vi "AlliGator Load IRFs & Fit Data (Map) HDF5 File v0.3.vi"(8 "Error In":errorcluster, 9 "File Type & Version only":bool, 11 "File Path":path) -> (0 "error out":errorcluster, 1 "Data Description":string, 2 "Decay Fit Options & Parameters":T1 {"Fit Options"."Offset Resolution" min=0.0; "Fit Options"."Period" min=0.0; "Fit Options"."Min Decay Percentile" min=0.0 max=1.0; "Fit Options"."Max Decay Percentile" min=0.0 max=100.0; "Fit Parameter Constraints"."Max Value" format="%#.3g"; "Fit Parameter Constraints"."Min Value" format="%#.3g"}, 3 "IRFs & Fit Data Map":T13 {"Fit Options: Decay Preprocessing Parameters"."# Folds" min=1}, 4 "[Multiple Decays Fit Parameters SDV]":dbl[][](array[numeric]), 5 "File Version":string, 7 "File Type":string)   [LabVIEW 2021, in "AlliGator Decay Fit Parameter Map.lvlib"]
doc: "Loads Decay Fit Parameter Map and associated metadata."
uses:
  AlliGator Decay Fit Parameter Map.lvlib
  AlliGator IRFs & Fit Data v2.ctl
  Fits/IRF(X)PSED/Decay Fit Parameters & Derived Quantities List.ctl
  AlliGator Decay Preprocessing Parameters.ctl
  Graphs/XY Graph/XY Graph Plot Shift Parameters.ctl
  Graphs/XY Graph/XY Graph Plot Shift Method.ctl
  AlliGator Decay Fit Options & Parameters v2.ctl
  Fits/IRF(X)PSED/Decay Fit Options v2.ctl
  Fits/Decay Convolution/Decay Model.ctl
  Fits/Residual Type.ctl
  Fits/IRF(X)PSED/Fit Weights Type.ctl
  Fits/Non-linear Fitting Method v2.ctl
  Fits/Fit Calculation Method.ctl
  Fits/Non-linear Fitting Algorithm.ctl
  AlliGator Decay Fit Parameter Constraints 2.ctl
  Fits/IRF(X)PSED/Decay Fit Parameters In List.ctl
  Fits/IRF(X)PSED/MLE Baseline Offset Type.ctl
  Fits/IRF(X)PSED/Decay Fit Options v1.ctl
  Fits/Non-linear Fitting Method v1.ctl
  AlliGator IRFs & Fit Data v1.ctl
  AlliGator Decay Fit Options & Parameters v1.ctl
  <vilib>/addons/h5labview2/base/lib_path.vi
  <vilib>/addons/h5labview2/base/H5Equery.vi
  <vilib>/addons/h5labview2/base/hid_t.ctl
  <vilib>/addons/h5labview2/dataset/H5Dread.llb/H5Dread.xnode
  <vilib>/addons/h5labview2/file/H5F.lvlib
  <vilib>/addons/h5labview2/group/H5G.lvlib
  Time/Time.lvlib
  Fits/Fits.lvlib
  Strings/Strings.lvlib
  AlliGator Decay Fit.lvlib
  Graphs/XY Graph/XY Graph Add-Ons.lvlib
  AlliGator Decay Preprocessing.lvlib
panel:
  in  "Fit Parameter":T12(ring)
  out "elapsed (relative) seconds":dbl
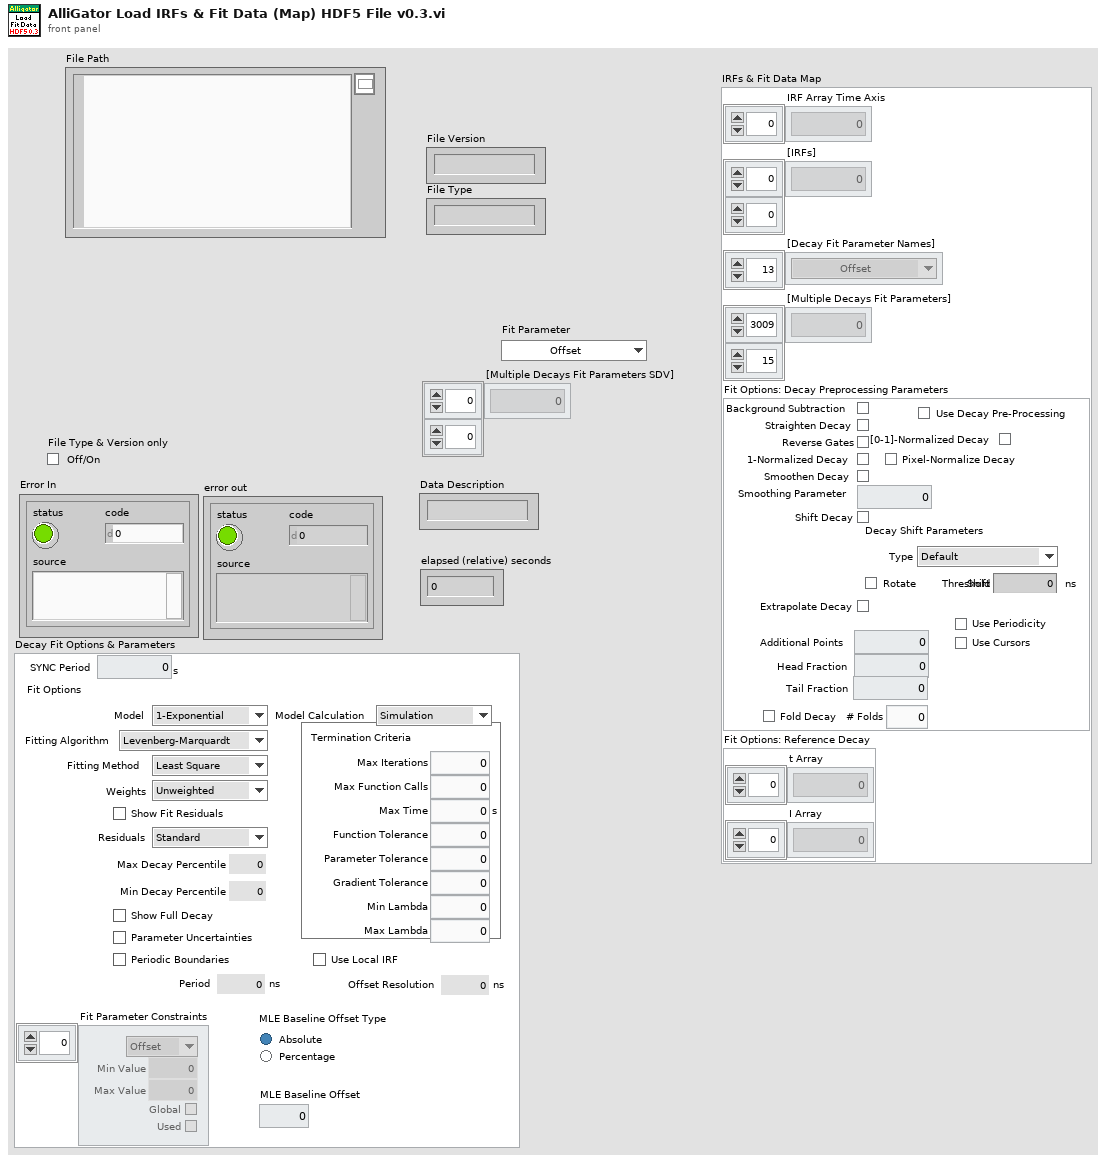
[diagram p1: front panel]
types:
  T1 = typedef "AlliGator Decay Fit Parameter Map.lvlib/AlliGator Decay Fit Options & Parameters v2.ctl" = cluster{"SYNC Period":dbl[unit], "Fit Options":T2, "Fit Parameter Constraints":T9[], "MLE Baseline Offset":dbl, "MLE Baseline Offset Type":T11}
  T2 = typedef "Fits.lvlib/Decay Fit Options v2.ctl" = cluster{"Show Fit Residuals":bool, "Fit Model":T3, "Residual Type":T4, "Max Decay Percentile":dbl, "Min Decay Percentile":dbl, "Show Full Decay":bool, "Weights":T5, "Fitting Method":T6, "Compute Parameter Uncertainties":bool, "Periodic Boundaries":bool, "Model Calculation":T7, "Period":dbl[unit], "Termination Criteria":cluster{"Max Iterations":i32, "Max Function Calls":i32, "Max Time":dbl[unit], "Function Tolerance":dbl, "Parameter Tolerance":dbl, "Gradient Tolerance":dbl, "Min Lambda":dbl, "Max Lambda":dbl, "Initial Tick Count":u32}, "Offset Resolution":dbl[unit], "Use Local IRF":bool, "Fitting Algorithm":T8}
  T3 = typedef "Fits.lvlib/Decay Model.ctl" = enum16{"1-Exponential", "2-Exponentials"}
  T4 = typedef "Fits.lvlib/Residual Type.ctl" = enum16{"Standard", "Normalized", "Reduced"}
  T5 = typedef "Fits.lvlib/Fit Weights Type.ctl" = enum16{"Unweighted", "1/Variance", "Best of All"}
  T6 = typedef "Fits.lvlib/Non-linear Fitting Method v2.ctl" = enum16{"Least Square", "Least Absolute Residual", "Bisquare", "MLE", "-", "Best of All"}
  T7 = typedef "Fits.lvlib/Fit Calculation Method.ctl" = enum16{"Simulation", "Convolution", "Integration"}
  T8 = typedef "Fits.lvlib/Non-linear Fitting Algorithm.ctl" = enum16{"Levenberg-Marquardt", "Trust-Region Dogleg"}
  T9 = typedef "AlliGator Decay Analysis.lvlib/AlliGator Decay Fit.lvlib/AlliGator Decay Fit Parameter Constraints 2.ctl" = cluster{"Fit Parameter":T10, "Min Value":dbl, "Max Value":dbl, "Global":bool, "Used":bool}
  T10 = typedef "Fits.lvlib/Decay Fit Parameters In List.ctl" = enum16{"Offset", "Baseline", "A_1", "tau_1", "A_2", "tau_2"}
  T11 = typedef "Fits.lvlib/MLE Baseline Offset Type.ctl" = enum32{"Absolute", "Percentage"}
  T12 = enum16{"Offset", "Baseline", "A_1", "tau_1", "A_2", "tau_2", "<tau>_1", "f1_1", "f2_1", "<tau>_2", "f1_2", "f2_2", "-", "R^2", "Chi^2"}
  T13 = typedef "AlliGator Decay Fit Parameter Map.lvlib/AlliGator IRFs & Fit Data v2.ctl" = cluster{"IRF Array Time Axis":dbl[], "[IRFs]":dbl[][], "[Decay Fit Parameter Names]":T14[], "[Multiple Decays Fit Parameters]":dbl[][], "Fit Options: Decay Preprocessing Parameters":T15, "Fit Options: Reference Decay":cluster{"t Array":dbl[], "I Array":dbl[]}}
  T14 = typedef "Fits.lvlib/Decay Fit Parameters & Derived Quantities List.ctl" = enum16{"Offset", "Baseline", "A_1", "tau_1", "A_2", "tau_2", "<tau>_a", "f1_a", "f2_a", "<tau>_i", "f1_i", "f2_i", "-", "R^2", "Chi^2"}
  T15 = typedef "AlliGator Decay Analysis.lvlib/AlliGator Decay Preprocessing.lvlib/AlliGator Decay Preprocessing Parameters.ctl" = cluster{"Background Subtraction":bool, "Straighten Decay":bool, "Reverse Gates":bool, "1-Normalized Decay":bool, "Smoothen Decay":bool, "Smoothing Parameter":dbl, "Shift Decay":bool, "Decay Shift Parameters":T16, "Extrapolate Decay":bool, "Additional Points":u32, "Head Fraction":dbl, "Pixel-Normalize Decay":bool, "Use Periodicity":bool, "Use Cursors":bool, "Tail Fraction":dbl, "Use Decay Pre-Processing":bool, "Fold Decay":bool, "# Folds":u32, "[0-1]-Normalized Decay":bool}
  T16 = typedef "XY Graph Add-Ons.lvlib/XY Graph Plot Shift Parameters.ctl" = cluster{"Type":T17, "Shift":dbl[unit], "Threshold":dbl, "Rotate":bool}
  T17 = typedef "XY Graph Add-Ons.lvlib/XY Graph Plot Shift Method.ctl" = enum16{"Default", "CFD", "Threshold", "Cross-Correlation"}
  T18 = typedef "AlliGator Decay Analysis.lvlib/AlliGator Decay Fit.lvlib/AlliGator Decay Fit Options & Parameters v1.ctl" = cluster{"SYNC Period":dbl[unit], "Fit Options":T19, "Fit Parameter Constraints":T9[]}
  T19 = typedef "Fits.lvlib/Decay Fit Options v1.ctl" = cluster{"Show Fit Residuals":bool, "Fit Model":T3, "Residual Type":T4, "Max Decay Percentile":dbl, "Min Decay Percentile":dbl, "Show Full Decay":bool, "Weights":T5, "Fitting Method":T20, "Compute Parameter Uncertainties":bool, "Periodic Boundaries":bool, "Model Calculation":T7, "Period":dbl[unit], "Termination Criteria":cluster{"Max Iterations":i32, "Max Function Calls":i32, "Max Time":dbl[unit], "Function Tolerance":dbl, "Parameter Tolerance":dbl, "Gradient Tolerance":dbl, "Min Lambda":dbl, "Max Lambda":dbl, "Initial Tick Count":u32}, "Offset Resolution":dbl[unit], "Use Local IRF":bool, "Fitting Algorithm":T8}
  T20 = typedef "Fits.lvlib/Non-linear Fitting Method v1.ctl" = enum16{"Least Square", "Least Absolute Residual", "Bisquare", "-", "Best of All"}
  T21 = typedef "AlliGator Decay Fit Parameter Map.lvlib/AlliGator IRFs & Fit Data v1.ctl" = cluster{"IRF Array Time Axis":dbl[], "[IRF]":dbl[][], "[Decay Fit Parameter Name]":T14[], "[Multiple Decays Fit Parameters]":dbl[][]}
  T22 = typedef "hid_t.ctl" = i64
  T23 = cluster{"Laser Period":dbl[unit], "Fit Options":T19, "Fit Parameter Constraints":T9[]}
  T24 = cluster{"IRF Array Time Axis":dbl[], "[IRF]":dbl[][], "[Decay Fit Parameter Name]":T14[], "[Multiple Decays Fit Parameters]":dbl[][]}
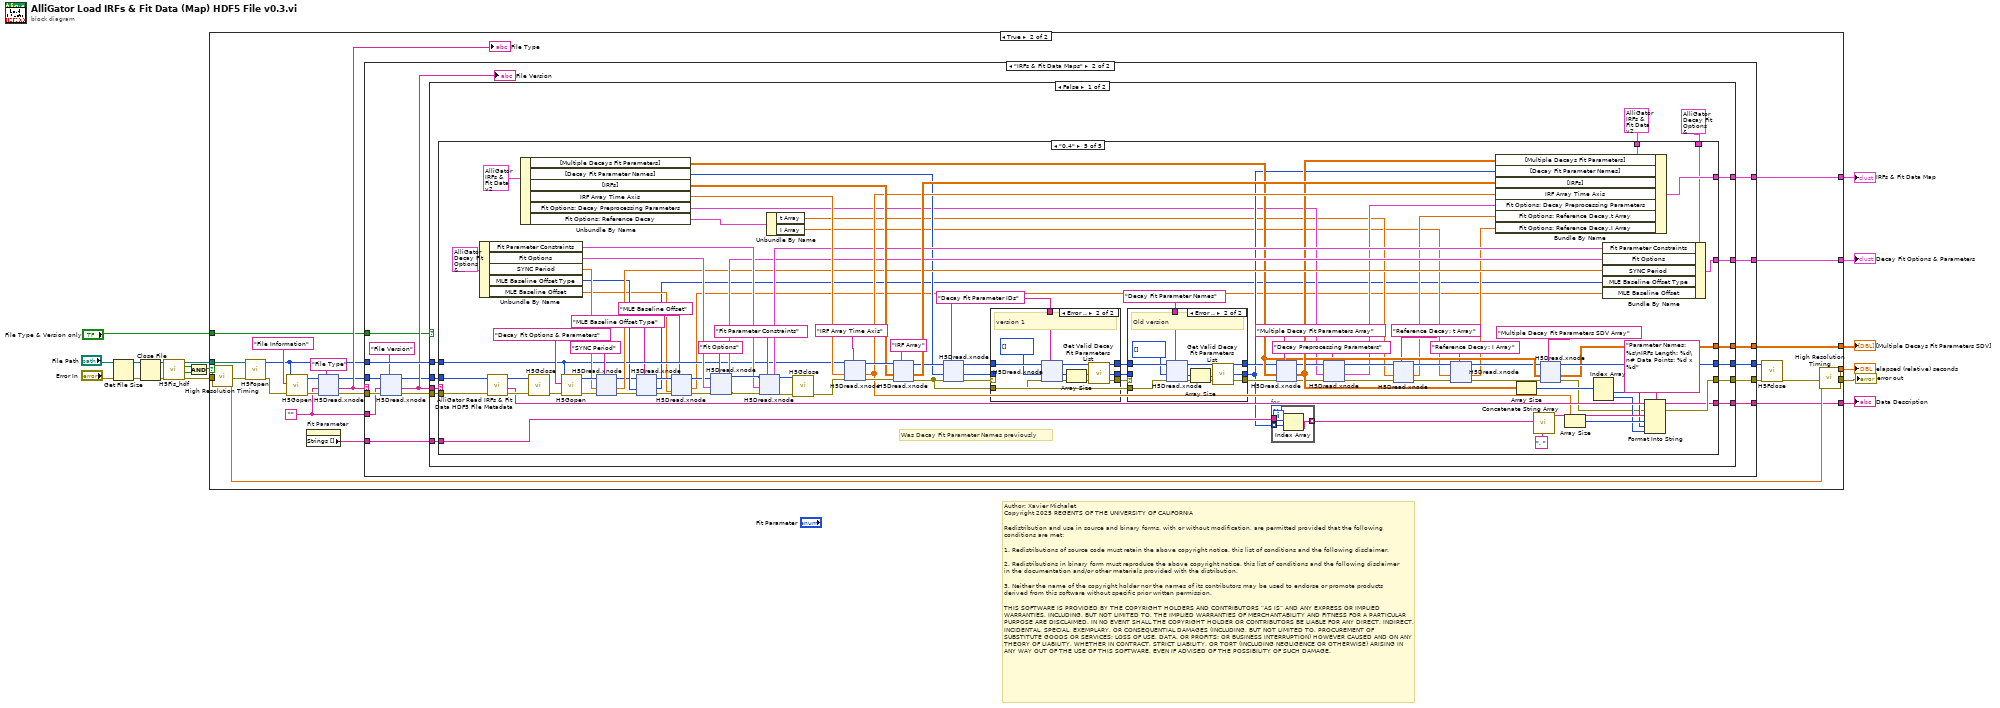
[diagram p0: block diagram]
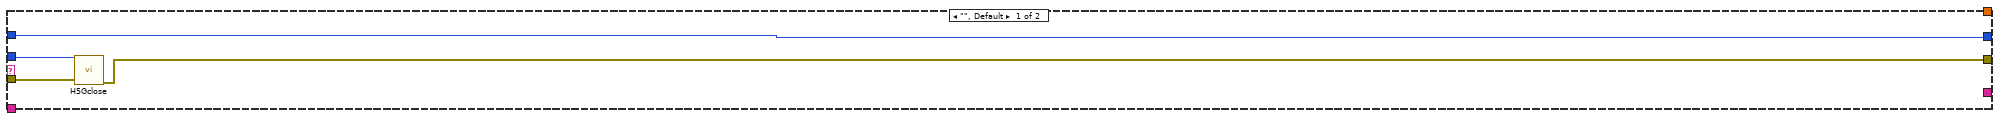
[diagram p3: hidden frame]
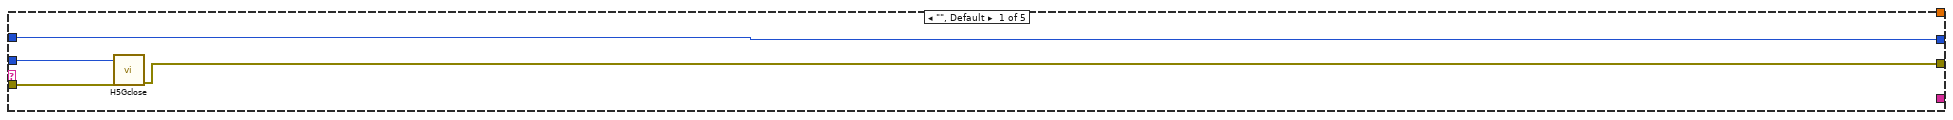
[diagram p4: hidden frame]
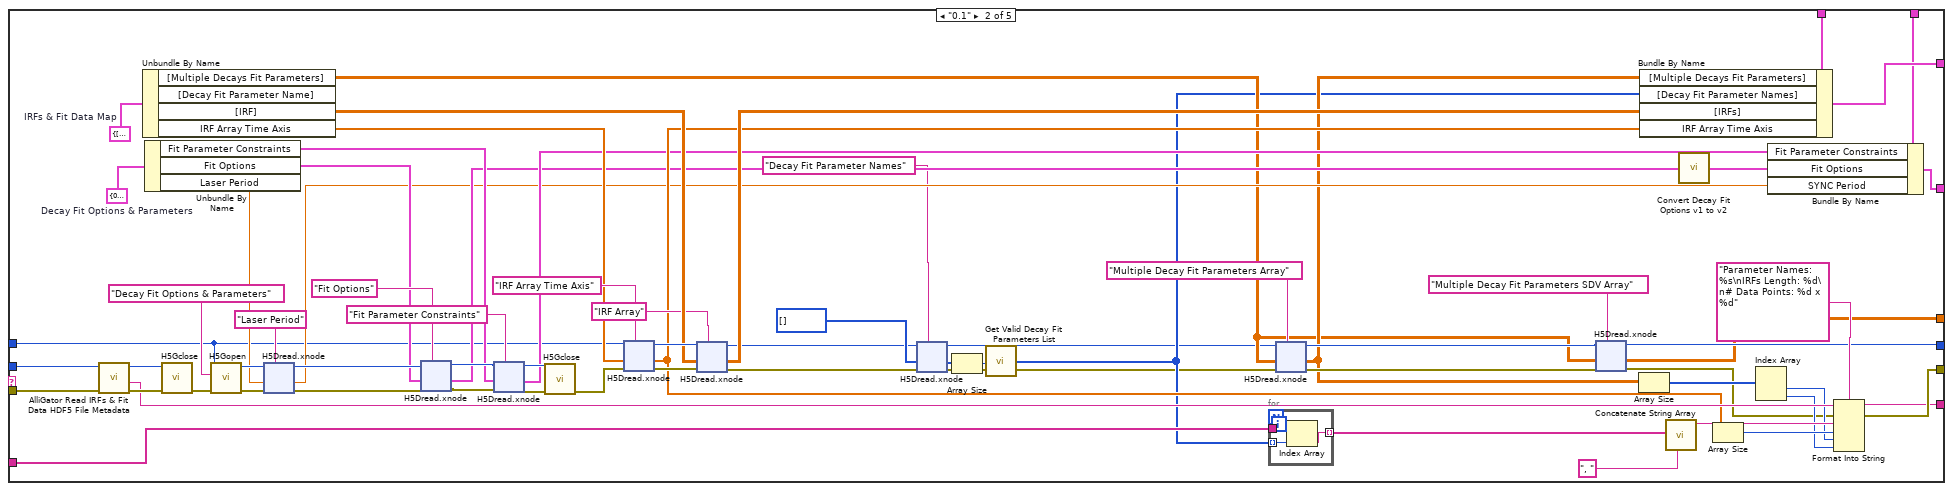
[diagram p5: hidden frame]
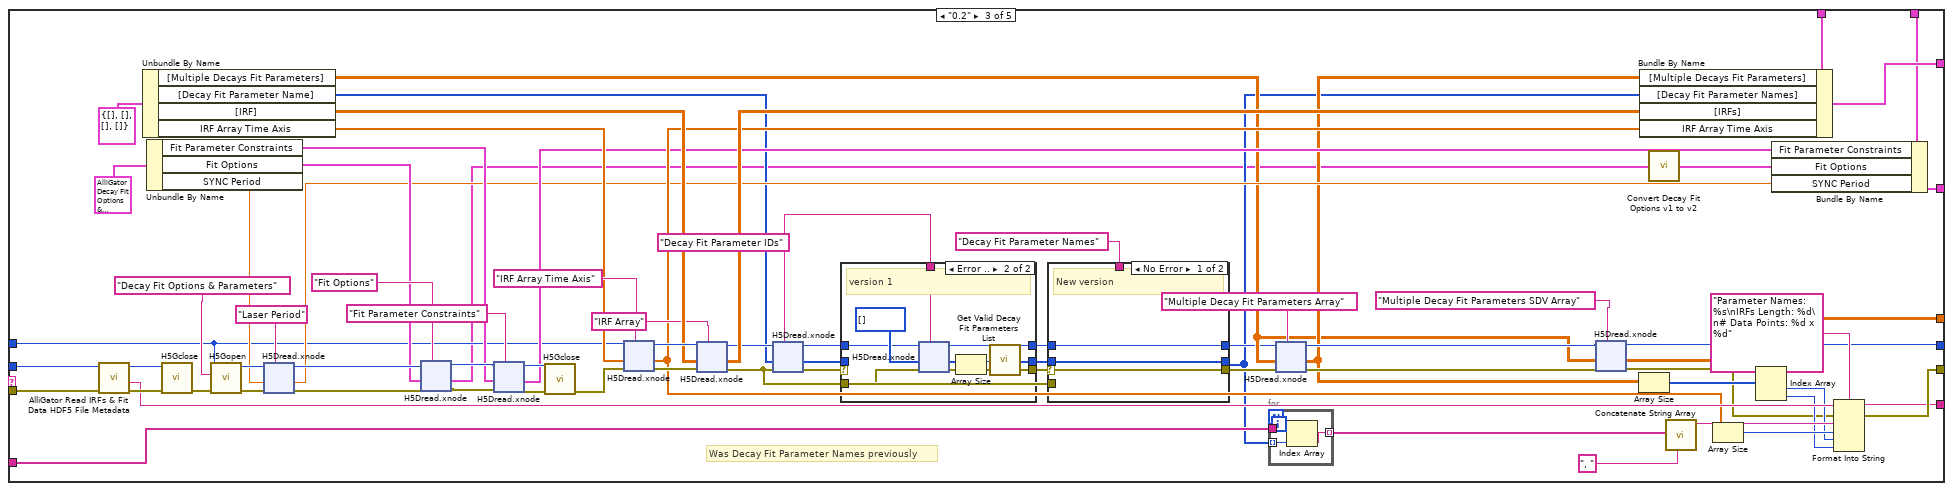
[diagram p6: hidden frame]
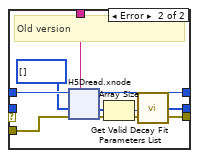
[diagram p8: hidden frame]
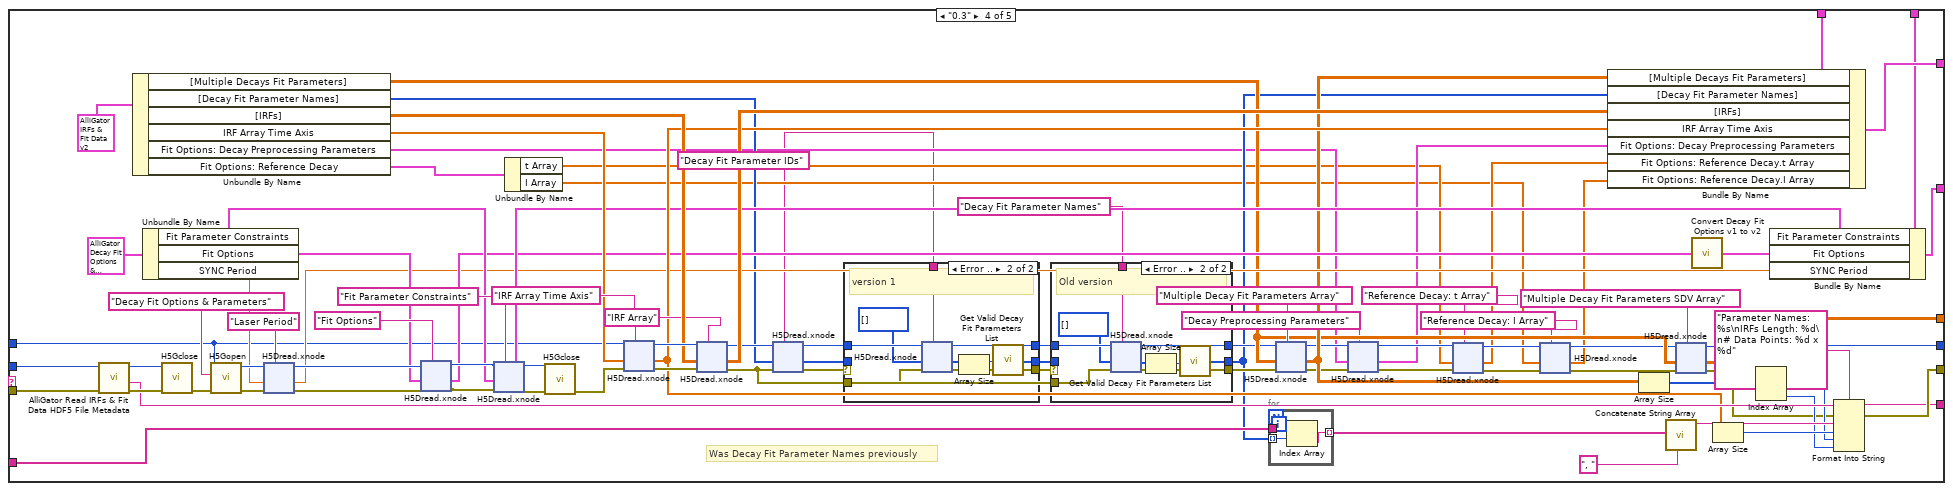
[diagram p9: hidden frame]
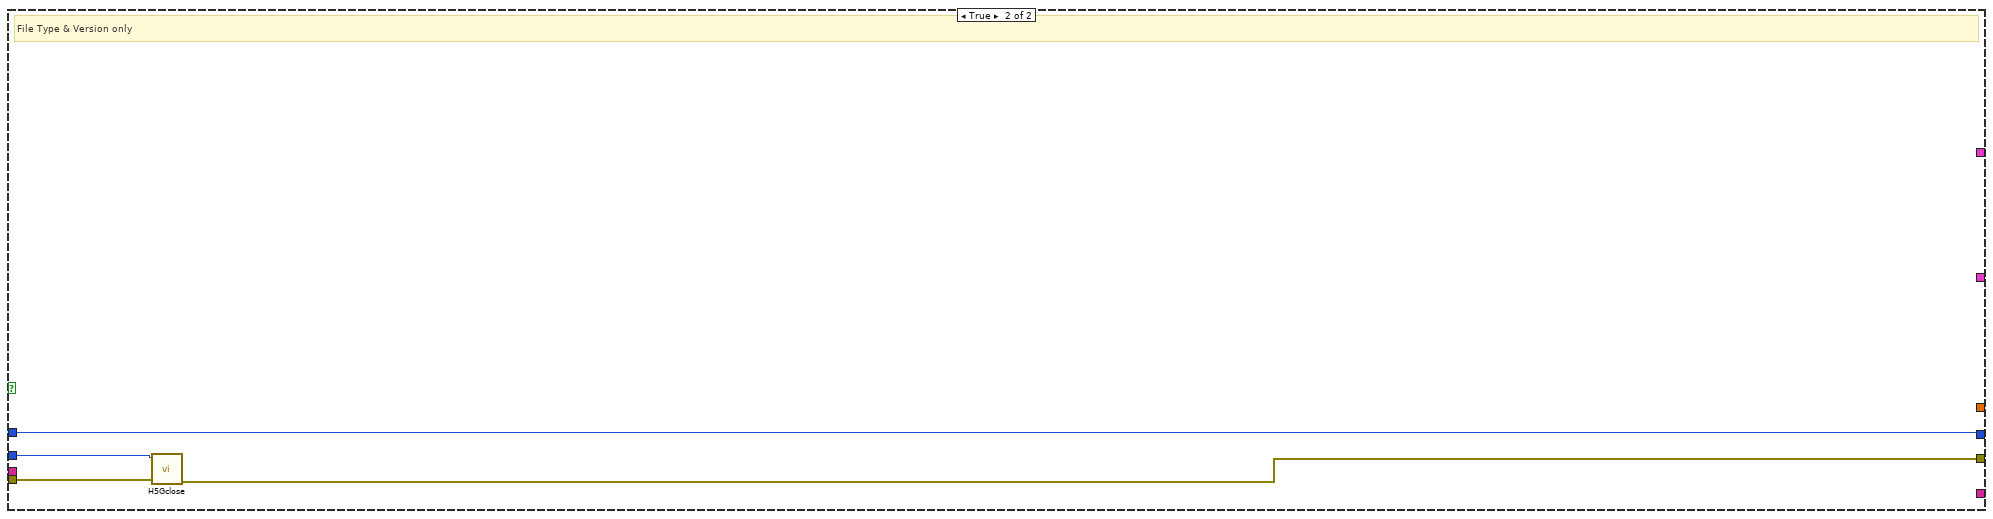
[diagram p14: hidden frame]
diagram:
  # "Author: Xavier Michalet\nCopyright 2025 REGENTS OF THE UNIVERSITY OF CALIFORNIA\n\nRedistribution and use in source and binary forms, with or without modification, are permitted provided that the following conditions are met:\n\n1. Redistributions of source code must retain the above copyright notice, this list of conditions and the following disclaimer.\n\n2. Redistributions in binary form must reproduce the above copyright notice, this list of conditions and the following disclaimer in the documentation and/or other materials provided with the distribution.\n\n3. Neither the name of the copyright holder nor the names of its contributors may be used to endorse or promote products derived from this software without specific prior written permission.\n\nTHIS SOFTWARE IS PROVIDED BY THE COPYRIGHT HOLDERS AND CONTRIBUTORS “AS IS” AND ANY EXPRESS OR IMPLIED WARRANTIES, INCLUDING, BUT NOT LIMITED TO, THE IMPLIED WARRANTIES OF MERCHANTABILITY AND FITNESS FOR A PARTICULAR PURPOSE ARE DISCLAIMED. IN NO EVENT SHALL THE COPYRIGHT HOLDER OR CONTRIBUTORS BE LIABLE FOR ANY DIRECT, INDIRECT, INCIDENTAL, SPECIAL, EXEMPLARY, OR CONSEQUENTIAL DAMAGES (INCLUDING, BUT NOT LIMITED TO, PROCUREMENT OF SUBSTITUTE GOODS OR SERVICES; LOSS OF USE, DATA, OR PROFITS; OR BUSINESS INTERRUPTION) HOWEVER CAUSED AND ON ANY THEORY OF LIABILITY, WHETHER IN CONTRACT, STRICT LIABILITY, OR TORT (INCLUDING NEGLIGENCE OR OTHERWISE) ARISING IN ANY WAY OUT OF THE USE OF THIS SOFTWARE, EVEN IF ADVISED OF THE POSSIBILITY OF SUCH DAMAGE."
  n1 = Get File Size(file="File Path", error in="Error In") -> (refnum out=w9:refnum<file>, 0:w10:errorcluster)  [unwired: 1 out]
  n2 = Close File(refnum=w9, error in=w10) -> (path=w8:path, error out=w7:errorcluster)
  n3 = call <vilib>:"H5Fis_hdf.vi"("error in (no error)"=w7, "path in"=w8) -> ("error out"=w14:errorcluster, "valid?"=w17:bool, "exists?"=w18:bool, "path out"=w15:path)  [unwired: 6 in]
  n4 = And(x=w18, y=w17) -> (x .and. y?=w16:bool)
  n5 = case shown="True" w16 {
    tunnel: w15 -> [_ w27]
    tunnel: w14 -> [w19 w44]
    tunnel: [w19 w39] -> w13
    tunnel: [_ w37] -> w6
    tunnel: [_ w26] -> w5
    tunnel: [_ w24] -> w4
    tunnel: [_ w22] -> w3
    tunnel: "File Type & Version only" -> [_ w21]
    tunnel: [_ w20] -> w1
    frame False {
    }
    frame True {
      w28 = ""
      n6 = call "High Resolution Timing.vi"("Error In"=w44) -> ("elapsed (relative) seconds"=w38:dbl, "Error Out"=w40:errorcluster)  [unwired: 16 in, 1 out]
      n7 = call <vilib>:"H5Fopen.vi"("error in (no error)"=w40, "path"=w27) -> ("error out"=w36:errorcluster, "ref out"=w31:T22)  [unwired: 8 in]
      n8 = call <vilib>:"H5Gopen.vi"("error in (no error)"=w36, "name"="File Information" ("dataset name (this)"), "ref in"=w31) -> ("error out"=w34:errorcluster, "group out"=w33:T22)  [unwired: 7 in]
      n9 = property on="Fit Parameter" class="Enum (strict)"() -> ("Strings []"=w23:string[])  [unwired: 2 in, 2 out]
      n10 = xnode "H5Dread.xnode"("dataset name (this)"="File Type", "error in (no error)"=w34, "default"=w28, "ref in"=w33) -> ("error out"=w30:errorcluster, "data"=w43:string, "ref out"=w29:T22)  [unwired: 2 in, 1 out]
      "File Type" <- w43
      n11 = case shown="\"IRFs & Fit Data Maps\"" w43 {
        tunnel: [w48 w64] -> w42
        tunnel: [w45 w57] -> w41
        tunnel: w31 -> [w48 w63]
        tunnel: w30 -> [w47 w61]
        tunnel: w28 -> [_ w60]
        tunnel: w29 -> [w46 w59]
        tunnel: [_ w56] -> w26
        tunnel: [_ w53] -> w24
        tunnel: w23 -> [_ w52]
        tunnel: [_ w51] -> w22
        tunnel: w21 -> [_ w50]
        tunnel: [_ w49] -> w20
        frame "", Default {
          n12 = call <vilib>:"H5Gclose.vi"("error in (no error)"=w47, "group in"=w46) -> ("error out"=w45:errorcluster)  [unwired: 9 in]
        }
        frame "IRFs & Fit Data Maps" {
          n13 = xnode "H5Dread.xnode"("dataset name (this)"="File Version", "error in (no error)"=w61, "default"=w60, "ref in"=w59) -> ("error out"=w55:errorcluster, "data"=w58:string, "ref out"=w54:T22)  [unwired: 2 in, 1 out]
          "File Version" <- w58
          n14 = case shown="False" w50 {
            tunnel: [w77 w1192] -> w64
            tunnel: w63 -> [w76 w1192]
            tunnel: w58 -> [w75 _]
            tunnel: [w74 w1191] -> w57
            tunnel: [w73 _] -> w56
            tunnel: w55 -> [w72 w1194]
            tunnel: w54 -> [w71 w1193]
            tunnel: [w70 _] -> w53
            tunnel: w52 -> [w69 _]
            tunnel: [w68 _] -> w51
            tunnel: [w67 _] -> w49
            frame False {
              n15 = case shown="\"0.4\"" w75 {
                tunnel: w76 -> [w81 w102 w300 w567 w890]
                tunnel: [w81 w98 w296 w565 w888] -> w77
                tunnel: [w78 w137 w334 w602 w923] -> w74
                tunnel: [_ w142 w339 w607 w928] -> w73
                tunnel: w72 -> [w80 w140 w337 w605 w926]
                tunnel: w71 -> [w79 w141 w338 w606 w927]
                tunnel: [_ w136 w333 w601 w922] -> w70
                tunnel: w69 -> [_ w133 w330 w598 w919]
                tunnel: [_ w103 w301 w568 w891] -> w68
                tunnel: [_ w94 w292 w561 w884] -> w67
                tunnel: T13 {"IRF Array Time Axis"=[], "[IRFs]"=[], "[Decay Fit Parameter Names]"=[], "[Multiple Decays Fit Parameters]"=[], "Fit Options: Decay Preprocessing Parameters"={"Background Subtraction"=FALSE, "Straighten Decay"=FALSE, "Reverse Gates"=FALSE, "1-Normalized Decay"=FALSE, "Smoothen Decay"=FALSE, "Smoothing Parameter"=0.0, "Shift Decay"=FALSE, "Decay Shift Parameters"={"Type"=enum."Default", "Shift"=0.0, "Threshold"=0.0, "Rotate"=FALSE}, "Extrapolate Decay"=FALSE, "Additional Points"=0, "Head Fraction"=0.0, "Pixel-Normalize Decay"=FALSE, "Use Periodicity"=FALSE, "Use Cursors"=FALSE, "Tail Fraction"=0.0, "Use Decay Pre-Processing"=FALSE, "Fold Decay"=FALSE, "# Folds"=0, "[0-1]-Normalized Decay"=FALSE}, "Fit Options: Reference Decay"={"t Array"=[], "I Array"=[]}} ("IRFs & Fit Data Map") -> [_ w93 w290 w555 w878]
                tunnel: T1 {"SYNC Period"=0.0, "Fit Options"={"Show Fit Residuals"=FALSE, "Fit Model"=enum."1-Exponential", "Residual Type"=enum."Standard", "Max Decay Percentile"=0.0, "Min Decay Percentile"=0.0, "Show Full Decay"=FALSE, "Weights"=enum."Unweighted", "Fitting Method"=enum."Least Square", "Compute Parameter Uncertainties"=FALSE, "Periodic Boundaries"=FALSE, "Model Calculation"=enum."Simulation", "Period"=0.0, "Termination Criteria"={"Max Iterations"=0, "Max Function Calls"=0, "Max Time"=0.0, "Function Tolerance"=0.0, "Parameter Tolerance"=0.0, "Gradient Tolerance"=0.0, "Min Lambda"=0.0, "Max Lambda"=0.0, "Initial Tick Count"=0}, "Offset Resolution"=0.0, "Use Local IRF"=FALSE, "Fitting Algorithm"=enum."Levenberg-Marquardt"}, "Fit Parameter Constraints"=[], "MLE Baseline Offset"=0.0, "MLE Baseline Offset Type"=enum."Absolute"} ("Decay Fit Options & Parameters") -> [_ w83 w277 w528 w851]
                frame "", Default {
                  n16 = call <vilib>:"H5Gclose.vi"("error in (no error)"=w80, "group in"=w79) -> ("error out"=w78:errorcluster)  [unwired: 9 in]
                }
                frame "0.1" {
                  w107 = T23 {"Laser Period"=0.0, "Fit Options"={"Show Fit Residuals"=FALSE, "Fit Model"=enum."1-Exponential", "Residual Type"=enum."Standard", "Max Decay Percentile"=0.0, "Min Decay Percentile"=0.0, "Show Full Decay"=FALSE, "Weights"=enum."Unweighted", "Fitting Method"=enum."Least Square", "Compute Parameter Uncertainties"=FALSE, "Periodic Boundaries"=FALSE, "Model Calculation"=enum."Simulation", "Period"=0.0, "Termination Criteria"={"Max Iterations"=0, "Max Function Calls"=0, "Max Time"=0.0, "Function Tolerance"=0.0, "Parameter Tolerance"=0.0, "Gradient Tolerance"=0.0, "Min Lambda"=0.0, "Max Lambda"=0.0, "Initial Tick Count"=0}, "Offset Resolution"=0.0, "Use Local IRF"=FALSE, "Fitting Algorithm"=enum."Levenberg-Marquardt"}, "Fit Parameter Constraints"=[]}  # Decay Fit Options & Parameters
                  w147 = T24 {"IRF Array Time Axis"=[], "[IRF]"=[], "[Decay Fit Parameter Name]"=[], "[Multiple Decays Fit Parameters]"=[]}  # IRFs & Fit Data Map
                  n17 = call "AlliGator Read IRFs & Fit Data HDF5 File Metadata.vi"("error in (no error)"=w140, "ref in"=w141) -> ("error out"=w138:errorcluster, "File Metadata"=w135:string, "ref out"=w139:T22)  [unwired: 7 in]
                  n18 = Unbundle By Name(w147) -> ("[Multiple Decays Fit Parameters]"=w95:dbl[][], "[IRF]"=w146:dbl[][], "IRF Array Time Axis"=w148:dbl[])  [unwired: 1 out]
                  n19 = Unbundle By Name(w107) -> ("Fit Parameter Constraints"=w108:T9[], "Fit Options"=w109:T19, "Laser Period"=w110:dbl[unit])
                  n20 = call <vilib>:"H5Gclose.vi"("error in (no error)"=w138, "group in"=w139) -> ("error out"=w113:errorcluster)  [unwired: 9 in]
                  n21 = call <vilib>:"H5Gopen.vi"("error in (no error)"=w113, "name"="Decay Fit Options & Parameters" ("dataset name"), "ref in"=w102) -> ("error out"=w124:errorcluster, "group out"=w123:T22)  [unwired: 7 in]
                  n22 = xnode "H5Dread.xnode"("dataset name (this)"="Laser Period" ("dataset name"), "error in (no error)"=w124, "default"=w110, "ref in"=w123) -> ("error out"=w122:errorcluster, "data"=w104:dbl[unit], "ref out"=w119:T22)  [unwired: 2 in, 1 out]
                  n23 = xnode "H5Dread.xnode"("dataset name (this)"="Fit Options" ("dataset name"), "error in (no error)"=w122, "default"=w109, "ref in"=w119) -> ("error out"=w121:errorcluster, "data"=w105:T19, "ref out"=w118:i64)  [unwired: 2 in, 1 out]
                  n24 = xnode "H5Dread.xnode"("dataset name (this)"="Fit Parameter Constraints" ("dataset name"), "error in (no error)"=w121, "default"=w108, "ref in"=w118) -> ("error out"=w120:errorcluster, "data"=w106:T9[], "ref out"=w117:i64)  [unwired: 2 in, 1 out]
                  n25 = call <vilib>:"H5Gclose.vi"("error in (no error)"=w120, "group in"=w117) -> ("error out"=w112:errorcluster)  [unwired: 9 in]
                  n26 = xnode "H5Dread.xnode"("dataset name (this)"="IRF Array Time Axis" ("dataset name"), "error in (no error)"=w112, "default"=w148, "ref in"=w102) -> ("error out"=w151:errorcluster, "data"=w128:dbl[], "ref out"=w150:T22)  [unwired: 2 in, 1 out]
                  n27 = xnode "H5Dread.xnode"("dataset name (this)"="IRF Array" ("dataset name"), "error in (no error)"=w151, "default"=w146, "ref in"=w150) -> ("error out"=w91:errorcluster, "data"=w144:dbl[][], "ref out"=w86:T22)  [unwired: 2 in, 1 out]
                  n28 = xnode "H5Dread.xnode"("dataset name (this)"="Decay Fit Parameter Names" ("name"), "error in (no error)"=w91, "default"=u16[] [], "ref in"=w86) -> ("error out"=w84:errorcluster, "data"=w89:u16[], "ref out"=w85:i64)  [unwired: 2 in, 1 out]
                  n29 = Array Size(array=w89) -> (size(s)=w88:i32)
                  n30 = call "Get Valid Decay Fit Parameters List.vi"("Parameter ID Array Size"=w88) -> ("Current Version"=w87:T14[])
                  n31 = for {
                    tunnel: w133 -> [w229]
                    tunnel: [w228] -> w132 mode=indexing
                    tunnel: w87 -> [w227] mode=indexing
                    n32 = Index Array(array=w229, index=w227) -> (element=w228:string)
                  }
                  n33 = xnode "H5Dread.xnode"("dataset name (this)"="Multiple Decay Fit Parameters Array" ("name"), "error in (no error)"=w84, "default"=w95, "ref in"=w85) -> ("error out"=w101:errorcluster, "data"=w96:dbl[][], "ref out"=w99:T22)  [unwired: 2 in, 1 out]
                  n34 = xnode "H5Dread.xnode"("dataset name (this)"="Multiple Decay Fit Parameters SDV Array" ("name"), "error in (no error)"=w101, "default"=w95, "ref in"=w99) -> ("error out"=w100:errorcluster, "data"=w94:dbl[][], "ref out"=w98:T22)  [unwired: 2 in, 1 out]
                  n35 = Array Size(array=w96) -> (size(s)=w127:i32[])
                  n36 = Bundle By Name(cluster=w93, "[Multiple Decays Fit Parameters]"=w96, "[Decay Fit Parameter Names]"=w87, "[IRFs]"=w144, "IRF Array Time Axis"=w128) -> (w142:T13)
                  n37 = call "Concatenate String Array.vi"("Separator (TAB)"=", ", "String Array"=w132) -> ("Formatted String"=w130:string)  [unwired: 9 in]
                  n38 = call "Convert Decay Fit Options v1 to v2.vi"("Decay Fit Options v1"=w105) -> ("Decay Fit Options v2"=w82:T2)
                  n39 = Array Size(array=w128) -> (size(s)=w129:i32)
                  n40 = Index Array(array=w127) -> (element #1=w126:i32, element #2=w125:i32)  [unwired: 2 in]
                  n41 = Bundle By Name(cluster=w83, "Fit Parameter Constraints"=w106, "Fit Options"=w82, "SYNC Period"=w104) -> (w103:T1)
                  n42 = Format Into String(format string="Parameter Names: %s\nIRFs Length: %d\n# Data Points: %d x %d", initial string=w135, error in=w100, w130, w129, w126, w125) -> (resulting string=w136:string, error out=w137:errorcluster)
                }
                frame "0.2" {
                  w285 = "Decay Fit Parameter IDs" ("name")
                  # "Was Decay Fit Parameter Names previously"
                  n43 = call "AlliGator Read IRFs & Fit Data HDF5 File Metadata.vi"("error in (no error)"=w337, "ref in"=w338) -> ("error out"=w335:errorcluster, "File Metadata"=w332:string, "ref out"=w336:T22)  [unwired: 7 in]
                  n44 = Unbundle By Name(T21 {"IRF Array Time Axis"=[], "[IRF]"=[], "[Decay Fit Parameter Name]"=[], "[Multiple Decays Fit Parameters]"=[]} ("IRFs & Fit Data Map")) -> ("[Multiple Decays Fit Parameters]"=w293:dbl[][], "[Decay Fit Parameter Name]"=w291:T14[], "[IRF]"=w344:dbl[][], "IRF Array Time Axis"=w346:dbl[])
                  n45 = Unbundle By Name(T18 {"SYNC Period"=0.0, "Fit Options"={"Show Fit Residuals"=FALSE, "Fit Model"=enum."1-Exponential", "Residual Type"=enum."Standard", "Max Decay Percentile"=0.0, "Min Decay Percentile"=0.0, "Show Full Decay"=FALSE, "Weights"=enum."Unweighted", "Fitting Method"=enum."Least Square", "Compute Parameter Uncertainties"=FALSE, "Periodic Boundaries"=FALSE, "Model Calculation"=enum."Simulation", "Period"=0.0, "Termination Criteria"={"Max Iterations"=0, "Max Function Calls"=0, "Max Time"=0.0, "Function Tolerance"=0.0, "Parameter Tolerance"=0.0, "Gradient Tolerance"=0.0, "Min Lambda"=0.0, "Max Lambda"=0.0, "Initial Tick Count"=0}, "Offset Resolution"=0.0, "Use Local IRF"=FALSE, "Fitting Algorithm"=enum."Levenberg-Marquardt"}, "Fit Parameter Constraints"=[]} ("Decay Fit Options & Parameters")) -> ("Fit Parameter Constraints"=w305:T9[], "Fit Options"=w306:T19, "SYNC Period"=w307:dbl[unit])
                  n46 = call <vilib>:"H5Gclose.vi"("error in (no error)"=w335, "group in"=w336) -> ("error out"=w310:errorcluster)  [unwired: 9 in]
                  n47 = call <vilib>:"H5Gopen.vi"("error in (no error)"=w310, "name"="Decay Fit Options & Parameters" ("dataset name"), "ref in"=w300) -> ("error out"=w321:errorcluster, "group out"=w320:T22)  [unwired: 7 in]
                  n48 = xnode "H5Dread.xnode"("dataset name (this)"="Laser Period" ("dataset name"), "error in (no error)"=w321, "default"=w307, "ref in"=w320) -> ("error out"=w319:errorcluster, "data"=w302:dbl[unit], "ref out"=w316:T22)  [unwired: 2 in, 1 out]
                  n49 = xnode "H5Dread.xnode"("dataset name (this)"="Fit Options" ("dataset name"), "error in (no error)"=w319, "default"=w306, "ref in"=w316) -> ("error out"=w318:errorcluster, "data"=w276:T19, "ref out"=w315:i64)  [unwired: 2 in, 1 out]
                  n50 = xnode "H5Dread.xnode"("dataset name (this)"="Fit Parameter Constraints" ("dataset name"), "error in (no error)"=w318, "default"=w305, "ref in"=w315) -> ("error out"=w317:errorcluster, "data"=w303:T9[], "ref out"=w314:T22)  [unwired: 2 in, 1 out]
                  n51 = call <vilib>:"H5Gclose.vi"("error in (no error)"=w317, "group in"=w314) -> ("error out"=w309:errorcluster)  [unwired: 9 in]
                  n52 = xnode "H5Dread.xnode"("dataset name (this)"="IRF Array Time Axis" ("dataset name"), "error in (no error)"=w309, "default"=w346, "ref in"=w300) -> ("error out"=w349:errorcluster, "data"=w325:dbl[], "ref out"=w348:T22)  [unwired: 2 in, 1 out]
                  n53 = xnode "H5Dread.xnode"("dataset name (this)"="IRF Array" ("dataset name"), "error in (no error)"=w349, "default"=w344, "ref in"=w348) -> ("error out"=w280:errorcluster, "data"=w342:dbl[][], "ref out"=w341:T22)  [unwired: 2 in, 1 out]
                  n54 = xnode "H5Dread.xnode"("dataset name (this)"=w285, "error in (no error)"=w280, "default"=w291, "ref in"=w341) -> ("error out"=w281:errorcluster, "data"=w279:T14[], "ref out"=w286:T22)  [unwired: 2 in, 1 out]
                  n55 = case shown="Error .." w281 {
                    selector: w281 -> [w352 _]
                    tunnel: [w351 w361] -> w289
                    tunnel: [w352 w360] -> w288
                    tunnel: [w350 w358] -> w287
                    tunnel: w286 -> [w351 w355]
                    tunnel: w285 -> [_ w354]
                    tunnel: w280 -> [_ w353]
                    tunnel: w279 -> [w350 _]
                    frame No Error {
                      # "New version"
                    }
                    frame Error {
                      # "version 1"
                      n56 = xnode "H5Dread.xnode"("dataset name (this)"=w354, "error in (no error)"=w353, "default"=u16[] [], "ref in"=w355) -> ("error out"=w360:errorcluster, "data"=w357:u16[], "ref out"=w361:i64)  [unwired: 2 in, 1 out]
                      n57 = Array Size(array=w357) -> (size(s)=w356:i32)
                      n58 = call "Get Valid Decay Fit Parameters List.vi"("Parameter ID Array Size"=w356) -> ("Current Version"=w358:T14[])
                    }
                  }
                  n59 = case shown="No Error" w288 {
                    selector: w288 -> [w378 _]
                    tunnel: w289 -> [w379 w388]
                    tunnel: [w379 w387] -> w282
                    tunnel: [w378 w386] -> w283
                    tunnel: w287 -> [w377 _]
                    tunnel: [w377 w385] -> w278
                    tunnel: "Decay Fit Parameter Names" ("name") -> [_ w381]
                    tunnel: w280 -> [_ w380]
                    frame No Error {
                      # "New version"
                    }
                    frame Error {
                      # "Old version"
                      n60 = xnode "H5Dread.xnode"("dataset name (this)"=w381, "error in (no error)"=w380, "default"=u16[] [], "ref in"=w388) -> ("error out"=w386:errorcluster, "data"=w383:u16[], "ref out"=w387:i64)  [unwired: 2 in, 1 out]
                      n61 = Array Size(array=w383) -> (size(s)=w382:i32)
                      n62 = call "Get Valid Decay Fit Parameters List.vi"("Parameter ID Array Size"=w382) -> ("Current Version"=w385:T14[])
                    }
                  }
                  n63 = for {
                    tunnel: w330 -> [w481]
                    tunnel: [w480] -> w329 mode=indexing
                    tunnel: w278 -> [w479] mode=indexing
                    n64 = Index Array(array=w481, index=w479) -> (element=w480:string)
                  }
                  n65 = xnode "H5Dread.xnode"("dataset name (this)"="Multiple Decay Fit Parameters Array" ("name"), "error in (no error)"=w283, "default"=w293, "ref in"=w282) -> ("error out"=w299:errorcluster, "data"=w294:dbl[][], "ref out"=w297:T22)  [unwired: 2 in, 1 out]
                  n66 = xnode "H5Dread.xnode"("dataset name (this)"="Multiple Decay Fit Parameters SDV Array" ("name"), "error in (no error)"=w299, "default"=w293, "ref in"=w297) -> ("error out"=w298:errorcluster, "data"=w292:dbl[][], "ref out"=w296:T22)  [unwired: 2 in, 1 out]
                  n67 = Array Size(array=w294) -> (size(s)=w324:i32[])
                  n68 = Bundle By Name(cluster=w290, "[Multiple Decays Fit Parameters]"=w294, "[Decay Fit Parameter Names]"=w278, "[IRFs]"=w342, "IRF Array Time Axis"=w325) -> (w339:T13)
                  n69 = call "Convert Decay Fit Options v1 to v2.vi"("Decay Fit Options v1"=w276) -> ("Decay Fit Options v2"=w275:T2)
                  n70 = call "Concatenate String Array.vi"("Separator (TAB)"=", ", "String Array"=w329) -> ("Formatted String"=w327:string)  [unwired: 9 in]
                  n71 = Array Size(array=w325) -> (size(s)=w326:i32)
                  n72 = Index Array(array=w324) -> (element #1=w323:i32, element #2=w322:i32)  [unwired: 2 in]
                  n73 = Bundle By Name(cluster=w277, "Fit Parameter Constraints"=w303, "Fit Options"=w275, "SYNC Period"=w302) -> (w301:T1)
                  n74 = Format Into String(format string="Parameter Names: %s\nIRFs Length: %d\n# Data Points: %d x %d", initial string=w332, error in=w298, w327, w326, w323, w322) -> (resulting string=w333:string, error out=w334:errorcluster)
                }
                frame "0.3" {
                  w535 = "Decay Fit Parameter IDs" ("name")
                  # "Was Decay Fit Parameter Names previously"
                  n75 = call "AlliGator Read IRFs & Fit Data HDF5 File Metadata.vi"("error in (no error)"=w605, "ref in"=w606) -> ("error out"=w603:errorcluster, "File Metadata"=w600:string, "ref out"=w604:T22)  [unwired: 7 in]
                  n76 = Unbundle By Name(T13 {"IRF Array Time Axis"=[], "[IRFs]"=[], "[Decay Fit Parameter Names]"=[], "[Multiple Decays Fit Parameters]"=[], "Fit Options: Decay Preprocessing Parameters"={"Background Subtraction"=FALSE, "Straighten Decay"=FALSE, "Reverse Gates"=FALSE, "1-Normalized Decay"=FALSE, "Smoothen Decay"=FALSE, "Smoothing Parameter"=0.0, "Shift Decay"=FALSE, "Decay Shift Parameters"={"Type"=enum."Default", "Shift"=0.0, "Threshold"=0.0, "Rotate"=FALSE}, "Extrapolate Decay"=FALSE, "Additional Points"=0, "Head Fraction"=0.0, "Pixel-Normalize Decay"=FALSE, "Use Periodicity"=FALSE, "Use Cursors"=FALSE, "Tail Fraction"=0.0, "Use Decay Pre-Processing"=FALSE, "Fold Decay"=FALSE, "# Folds"=0, "[0-1]-Normalized Decay"=FALSE}, "Fit Options: Reference Decay"={"t Array"=[], "I Array"=[]}} ("IRFs & Fit Data Map")) -> ("[Multiple Decays Fit Parameters]"=w562:dbl[][], "[Decay Fit Parameter Names]"=w556:T14[], "[IRFs]"=w612:dbl[][], "IRF Array Time Axis"=w614:dbl[], "Fit Options: Decay Preprocessing Parameters"=w543:T15, "Fit Options: Reference Decay"=w541:cluster{"t Array":dbl[], "I Array":dbl[]})
                  n77 = Unbundle By Name(T18 {"SYNC Period"=0.0, "Fit Options"={"Show Fit Residuals"=FALSE, "Fit Model"=enum."1-Exponential", "Residual Type"=enum."Standard", "Max Decay Percentile"=0.0, "Min Decay Percentile"=0.0, "Show Full Decay"=FALSE, "Weights"=enum."Unweighted", "Fitting Method"=enum."Least Square", "Compute Parameter Uncertainties"=FALSE, "Periodic Boundaries"=FALSE, "Model Calculation"=enum."Simulation", "Period"=0.0, "Termination Criteria"={"Max Iterations"=0, "Max Function Calls"=0, "Max Time"=0.0, "Function Tolerance"=0.0, "Parameter Tolerance"=0.0, "Gradient Tolerance"=0.0, "Min Lambda"=0.0, "Max Lambda"=0.0, "Initial Tick Count"=0}, "Offset Resolution"=0.0, "Use Local IRF"=FALSE, "Fitting Algorithm"=enum."Levenberg-Marquardt"}, "Fit Parameter Constraints"=[]} ("Decay Fit Options & Parameters")) -> ("Fit Parameter Constraints"=w573:T9[], "Fit Options"=w574:T19, "SYNC Period"=w575:dbl[unit])
                  n78 = call <vilib>:"H5Gclose.vi"("error in (no error)"=w603, "group in"=w604) -> ("error out"=w578:errorcluster)  [unwired: 9 in]
                  n79 = call <vilib>:"H5Gopen.vi"("error in (no error)"=w578, "name"="Decay Fit Options & Parameters" ("dataset name"), "ref in"=w567) -> ("error out"=w589:errorcluster, "group out"=w588:T22)  [unwired: 7 in]
                  n80 = xnode "H5Dread.xnode"("dataset name (this)"="Laser Period" ("dataset name"), "error in (no error)"=w589, "default"=w575, "ref in"=w588) -> ("error out"=w587:errorcluster, "data"=w569:dbl[unit], "ref out"=w584:T22)  [unwired: 2 in, 1 out]
                  n81 = xnode "H5Dread.xnode"("dataset name (this)"="Fit Options" ("dataset name"), "error in (no error)"=w587, "default"=w574, "ref in"=w584) -> ("error out"=w586:errorcluster, "data"=w570:T19, "ref out"=w583:i64)  [unwired: 2 in, 1 out]
                  n82 = xnode "H5Dread.xnode"("dataset name (this)"="Fit Parameter Constraints" ("dataset name"), "error in (no error)"=w586, "default"=w573, "ref in"=w583) -> ("error out"=w585:errorcluster, "data"=w571:T9[], "ref out"=w582:T22)  [unwired: 2 in, 1 out]
                  n83 = Unbundle By Name(w541) -> ("t Array"=w540:dbl[], "I Array"=w538:dbl[])
                  n84 = call <vilib>:"H5Gclose.vi"("error in (no error)"=w585, "group in"=w582) -> ("error out"=w577:errorcluster)  [unwired: 9 in]
                  n85 = xnode "H5Dread.xnode"("dataset name (this)"="IRF Array Time Axis" ("dataset name"), "error in (no error)"=w577, "default"=w614, "ref in"=w567) -> ("error out"=w617:errorcluster, "data"=w593:dbl[], "ref out"=w616:T22)  [unwired: 2 in, 1 out]
                  n86 = xnode "H5Dread.xnode"("dataset name (this)"="IRF Array" ("dataset name"), "error in (no error)"=w617, "default"=w612, "ref in"=w616) -> ("error out"=w530:errorcluster, "data"=w610:dbl[][], "ref out"=w609:T22)  [unwired: 2 in, 1 out]
                  n87 = xnode "H5Dread.xnode"("dataset name (this)"=w535, "error in (no error)"=w530, "default"=w556, "ref in"=w609) -> ("error out"=w536:errorcluster, "data"=w533:T14[], "ref out"=w532:T22)  [unwired: 2 in, 1 out]
                  n88 = case shown="Error .." w536 {
                    selector: w536 -> [w619 _]
                    tunnel: w532 -> [w620 w625]
                    tunnel: [w620 w629] -> w534
                    tunnel: [w619 w627] -> w531
                    tunnel: [w618 w623] -> w529
                    tunnel: w535 -> [_ w628]
                    tunnel: w530 -> [_ w626]
                    tunnel: w533 -> [w618 _]
                    frame No Error {
                      # "New version"
                    }
                    frame Error {
                      # "version 1"
                      n89 = xnode "H5Dread.xnode"("dataset name (this)"=w628, "error in (no error)"=w626, "default"=u16[] [], "ref in"=w625) -> ("error out"=w627:errorcluster, "data"=w622:u16[], "ref out"=w629:i64)  [unwired: 2 in, 1 out]
                      n90 = Array Size(array=w622) -> (size(s)=w621:i32)
                      n91 = call "Get Valid Decay Fit Parameters List.vi"("Parameter ID Array Size"=w621) -> ("Current Version"=w623:T14[])
                    }
                  }
                  n92 = case shown="Error .." w531 {
                    selector: w531 -> [w691 _]
                    tunnel: w534 -> [w692 w701]
                    tunnel: [w692 w700] -> w560
                    tunnel: [w691 w698] -> w559
                    tunnel: w529 -> [w690 _]
                    tunnel: [w690 w696] -> w558
                    tunnel: "Decay Fit Parameter Names" ("name") -> [_ w699]
                    tunnel: w530 -> [_ w697]
                    frame No Error {
                      # "New version"
                    }
                    frame Error {
                      # "Old version"
                      n93 = xnode "H5Dread.xnode"("dataset name (this)"=w699, "error in (no error)"=w697, "default"=u16[] [], "ref in"=w701) -> ("error out"=w698:errorcluster, "data"=w694:u16[], "ref out"=w700:i64)  [unwired: 2 in, 1 out]
                      n94 = Array Size(array=w694) -> (size(s)=w693:i32)
                      n95 = call "Get Valid Decay Fit Parameters List.vi"("Parameter ID Array Size"=w693) -> ("Current Version"=w696:T14[])
                    }
                  }
                  n96 = for {
                    tunnel: w558 -> [w778] mode=indexing
                    tunnel: w598 -> [w779]
                    tunnel: [w777] -> w597 mode=indexing
                    n97 = Index Array(array=w779, index=w778) -> (element=w777:string)
                  }
                  n98 = xnode "H5Dread.xnode"("dataset name (this)"="Multiple Decay Fit Parameters Array" ("name"), "error in (no error)"=w559, "default"=w562, "ref in"=w560) -> ("error out"=w553:errorcluster, "data"=w563:dbl[][], "ref out"=w554:T22)  [unwired: 2 in, 1 out]
                  n99 = xnode "H5Dread.xnode"("dataset name (this)"="Decay Preprocessing Parameters" ("name"), "error in (no error)"=w553, "default"=w543, "ref in"=w554) -> ("error out"=w549:errorcluster, "data"=w542:T15, "ref out"=w552:i64)  [unwired: 2 in, 1 out]
                  n100 = xnode "H5Dread.xnode"("dataset name (this)"="Reference Decay: t Array" ("name"), "error in (no error)"=w549, "default"=w540, "ref in"=w552) -> ("error out"=w548:errorcluster, "data"=w539:dbl[], "ref out"=w551:T22)  [unwired: 2 in, 1 out]
                  n101 = xnode "H5Dread.xnode"("dataset name (this)"="Reference Decay: I Array" ("name"), "error in (no error)"=w548, "default"=w538, "ref in"=w551) -> ("error out"=w547:errorcluster, "data"=w537:dbl[], "ref out"=w550:T22)  [unwired: 2 in, 1 out]
                  n102 = Bundle By Name(cluster=w555, "[Multiple Decays Fit Parameters]"=w563, "[Decay Fit Parameter Names]"=w558, "[IRFs]"=w610, "IRF Array Time Axis"=w593, "Fit Options: Decay Preprocessing Parameters"=w542, "Fit Options: Reference Decay.t Array"=w539, "Fit Options: Reference Decay.I Array"=w537) -> (w607:T13)
                  n103 = Array Size(array=w563) -> (size(s)=w592:i32[])
                  n104 = call "Concatenate String Array.vi"("Separator (TAB)"=", ", "String Array"=w597) -> ("Formatted String"=w595:string)  [unwired: 9 in]
                  n105 = xnode "H5Dread.xnode"("dataset name (this)"="Multiple Decay Fit Parameters SDV Array" ("name"), "error in (no error)"=w547, "default"=w562, "ref in"=w550) -> ("error out"=w566:errorcluster, "data"=w561:dbl[][], "ref out"=w565:T22)  [unwired: 2 in, 1 out]
                  n106 = call "Convert Decay Fit Options v1 to v2.vi"("Decay Fit Options v1"=w570) -> ("Decay Fit Options v2"=w527:T2)
                  n107 = Array Size(array=w593) -> (size(s)=w594:i32)
                  n108 = Index Array(array=w592) -> (element #1=w591:i32, element #2=w590:i32)  [unwired: 2 in]
                  n109 = Bundle By Name(cluster=w528, "Fit Parameter Constraints"=w571, "Fit Options"=w527, "SYNC Period"=w569) -> (w568:T1)
                  n110 = Format Into String(format string="Parameter Names: %s\nIRFs Length: %d\n# Data Points: %d x %d", initial string=w600, error in=w566, w595, w594, w591, w590) -> (resulting string=w601:string, error out=w602:errorcluster)
                }
                frame "0.4" {
                  w858 = "Decay Fit Parameter IDs" ("name")
                  # "Was Decay Fit Parameter Names previously"
                  n111 = Unbundle By Name(T1 {"SYNC Period"=0.0, "Fit Options"={"Show Fit Residuals"=FALSE, "Fit Model"=enum."1-Exponential", "Residual Type"=enum."Standard", "Max Decay Percentile"=0.0, "Min Decay Percentile"=0.0, "Show Full Decay"=FALSE, "Weights"=enum."Unweighted", "Fitting Method"=enum."Least Square", "Compute Parameter Uncertainties"=FALSE, "Periodic Boundaries"=FALSE, "Model Calculation"=enum."Simulation", "Period"=0.0, "Termination Criteria"={"Max Iterations"=0, "Max Function Calls"=0, "Max Time"=0.0, "Function Tolerance"=0.0, "Parameter Tolerance"=0.0, "Gradient Tolerance"=0.0, "Min Lambda"=0.0, "Max Lambda"=0.0, "Initial Tick Count"=0}, "Offset Resolution"=0.0, "Use Local IRF"=FALSE, "Fitting Algorithm"=enum."Levenberg-Marquardt"}, "Fit Parameter Constraints"=[], "MLE Baseline Offset"=0.0, "MLE Baseline Offset Type"=enum."Absolute"} ("Decay Fit Options & Parameters")) -> ("Fit Parameter Constraints"=w896:T9[], "Fit Options"=w897:T2, "SYNC Period"=w898:dbl[unit], "MLE Baseline Offset Type"=w848:T11, "MLE Baseline Offset"=w842:dbl)
                  n112 = call "AlliGator Read IRFs & Fit Data HDF5 File Metadata.vi"("error in (no error)"=w926, "ref in"=w927) -> ("error out"=w924:errorcluster, "File Metadata"=w921:string, "ref out"=w925:T22)  [unwired: 7 in]
                  n113 = Unbundle By Name(T13 {"IRF Array Time Axis"=[], "[IRFs]"=[], "[Decay Fit Parameter Names]"=[], "[Multiple Decays Fit Parameters]"=[], "Fit Options: Decay Preprocessing Parameters"={"Background Subtraction"=FALSE, "Straighten Decay"=FALSE, "Reverse Gates"=FALSE, "1-Normalized Decay"=FALSE, "Smoothen Decay"=FALSE, "Smoothing Parameter"=0.0, "Shift Decay"=FALSE, "Decay Shift Parameters"={"Type"=enum."Default", "Shift"=0.0, "Threshold"=0.0, "Rotate"=FALSE}, "Extrapolate Decay"=FALSE, "Additional Points"=0, "Head Fraction"=0.0, "Pixel-Normalize Decay"=FALSE, "Use Periodicity"=FALSE, "Use Cursors"=FALSE, "Tail Fraction"=0.0, "Use Decay Pre-Processing"=FALSE, "Fold Decay"=FALSE, "# Folds"=0, "[0-1]-Normalized Decay"=FALSE}, "Fit Options: Reference Decay"={"t Array"=[], "I Array"=[]}} ("IRFs & Fit Data Map")) -> ("[Multiple Decays Fit Parameters]"=w885:dbl[][], "[Decay Fit Parameter Names]"=w879:T14[], "[IRFs]"=w933:dbl[][], "IRF Array Time Axis"=w935:dbl[], "Fit Options: Decay Preprocessing Parameters"=w866:T15, "Fit Options: Reference Decay"=w864:cluster{"t Array":dbl[], "I Array":dbl[]})
                  n114 = call <vilib>:"H5Gclose.vi"("error in (no error)"=w924, "group in"=w925) -> ("error out"=w901:errorcluster)  [unwired: 9 in]
                  n115 = call <vilib>:"H5Gopen.vi"("error in (no error)"=w901, "name"="Decay Fit Options & Parameters" ("dataset name"), "ref in"=w890) -> ("error out"=w910:errorcluster, "group out"=w909:T22)  [unwired: 7 in]
                  n116 = xnode "H5Dread.xnode"("dataset name (this)"="SYNC Period" ("dataset name"), "error in (no error)"=w910, "default"=w898, "ref in"=w909) -> ("error out"=w850:errorcluster, "data"=w892:dbl[unit], "ref out"=w847:T22)  [unwired: 2 in, 1 out]
                  n117 = xnode "H5Dread.xnode"("dataset name (this)"="MLE Baseline Offset Type" ("dataset name"), "error in (no error)"=w850, "default"=w848, "ref in"=w847) -> ("error out"=w846:errorcluster, "data"=w841:T11)  [unwired: 2 in, 2 out]
                  n118 = xnode "H5Dread.xnode"("dataset name (this)"="MLE Baseline Offset" ("dataset name"), "error in (no error)"=w846, "default"=w842, "ref in"=w847) -> ("error out"=w844:errorcluster, "data"=w840:dbl, "ref out"=w845:i64)  [unwired: 2 in, 1 out]
                  n119 = xnode "H5Dread.xnode"("dataset name (this)"="Fit Options" ("dataset name"), "error in (no error)"=w844, "default"=w897, "ref in"=w845) -> ("error out"=w908:errorcluster, "data"=w893:T2, "ref out"=w906:i64)  [unwired: 2 in, 1 out]
                  n120 = xnode "H5Dread.xnode"("dataset name (this)"="Fit Parameter Constraints" ("dataset name"), "error in (no error)"=w908, "default"=w896, "ref in"=w906) -> ("error out"=w907:errorcluster, "data"=w894:T9[], "ref out"=w905:T22)  [unwired: 2 in, 1 out]
                  n121 = Unbundle By Name(w864) -> ("t Array"=w863:dbl[], "I Array"=w861:dbl[])
                  n122 = call <vilib>:"H5Gclose.vi"("error in (no error)"=w907, "group in"=w905) -> ("error out"=w900:errorcluster)  [unwired: 9 in]
                  n123 = xnode "H5Dread.xnode"("dataset name (this)"="IRF Array Time Axis" ("dataset name"), "error in (no error)"=w900, "default"=w935, "ref in"=w890) -> ("error out"=w938:errorcluster, "data"=w914:dbl[], "ref out"=w937:T22)  [unwired: 2 in, 1 out]
                  n124 = xnode "H5Dread.xnode"("dataset name (this)"="IRF Array" ("dataset name"), "error in (no error)"=w938, "default"=w933, "ref in"=w937) -> ("error out"=w853:errorcluster, "data"=w931:dbl[][], "ref out"=w930:T22)  [unwired: 2 in, 1 out]
                  n125 = xnode "H5Dread.xnode"("dataset name (this)"=w858, "error in (no error)"=w853, "default"=w879, "ref in"=w930) -> ("error out"=w859:errorcluster, "data"=w856:T14[], "ref out"=w855:T22)  [unwired: 2 in, 1 out]
                  n126 = case shown="Error .." w859 {
                    selector: w859 -> [w970 _]
                    tunnel: w855 -> [w971 w976]
                    tunnel: [w971 w980] -> w857
                    tunnel: [w970 w978] -> w854
                    tunnel: [w969 w974] -> w852
                    tunnel: w858 -> [_ w979]
                    tunnel: w853 -> [_ w977]
                    tunnel: w856 -> [w969 _]
                    frame No Error {
                      # "New version"
                    }
                    frame Error {
                      # "version 1"
                      n127 = xnode "H5Dread.xnode"("dataset name (this)"=w979, "error in (no error)"=w977, "default"=u16[] [], "ref in"=w976) -> ("error out"=w978:errorcluster, "data"=w973:u16[], "ref out"=w980:i64)  [unwired: 2 in, 1 out]
                      n128 = Array Size(array=w973) -> (size(s)=w972:i32)
                      n129 = call "Get Valid Decay Fit Parameters List.vi"("Parameter ID Array Size"=w972) -> ("Current Version"=w974:T14[])
                    }
                  }
                  n130 = case shown="Error .." w854 {
                    selector: w854 -> [w1042 _]
                    tunnel: w857 -> [w1043 w1052]
                    tunnel: [w1043 w1051] -> w883
                    tunnel: [w1042 w1049] -> w882
                    tunnel: w852 -> [w1041 _]
                    tunnel: [w1041 w1047] -> w881
                    tunnel: "Decay Fit Parameter Names" ("name") -> [_ w1050]
                    tunnel: w853 -> [_ w1048]
                    frame No Error {
                      # "New version"
                    }
                    frame Error {
                      # "Old version"
                      n131 = xnode "H5Dread.xnode"("dataset name (this)"=w1050, "error in (no error)"=w1048, "default"=u16[] [], "ref in"=w1052) -> ("error out"=w1049:errorcluster, "data"=w1045:u16[], "ref out"=w1051:i64)  [unwired: 2 in, 1 out]
                      n132 = Array Size(array=w1045) -> (size(s)=w1044:i32)
                      n133 = call "Get Valid Decay Fit Parameters List.vi"("Parameter ID Array Size"=w1044) -> ("Current Version"=w1047:T14[])
                    }
                  }
                  n134 = for {
                    tunnel: w881 -> [w1129] mode=indexing
                    tunnel: w919 -> [w1130]
                    tunnel: [w1128] -> w918 mode=indexing
                    n135 = Index Array(array=w1130, index=w1129) -> (element=w1128:string)
                  }
                  n136 = xnode "H5Dread.xnode"("dataset name (this)"="Multiple Decay Fit Parameters Array" ("name"), "error in (no error)"=w882, "default"=w885, "ref in"=w883) -> ("error out"=w876:errorcluster, "data"=w886:dbl[][], "ref out"=w877:T22)  [unwired: 2 in, 1 out]
                  n137 = xnode "H5Dread.xnode"("dataset name (this)"="Decay Preprocessing Parameters" ("name"), "error in (no error)"=w876, "default"=w866, "ref in"=w877) -> ("error out"=w872:errorcluster, "data"=w865:T15, "ref out"=w875:T22)  [unwired: 2 in, 1 out]
                  n138 = xnode "H5Dread.xnode"("dataset name (this)"="Reference Decay: t Array" ("name"), "error in (no error)"=w872, "default"=w863, "ref in"=w875) -> ("error out"=w871:errorcluster, "data"=w862:dbl[], "ref out"=w874:T22)  [unwired: 2 in, 1 out]
                  n139 = xnode "H5Dread.xnode"("dataset name (this)"="Reference Decay: I Array" ("name"), "error in (no error)"=w871, "default"=w861, "ref in"=w874) -> ("error out"=w870:errorcluster, "data"=w860:dbl[], "ref out"=w873:T22)  [unwired: 2 in, 1 out]
                  n140 = Bundle By Name(cluster=w878, "[Multiple Decays Fit Parameters]"=w886, "[Decay Fit Parameter Names]"=w881, "[IRFs]"=w931, "IRF Array Time Axis"=w914, "Fit Options: Decay Preprocessing Parameters"=w865, "Fit Options: Reference Decay.t Array"=w862, "Fit Options: Reference Decay.I Array"=w860) -> (w928:T13)
                  n141 = Array Size(array=w886) -> (size(s)=w913:i32[])
                  n142 = call "Concatenate String Array.vi"("Separator (TAB)"=", ", "String Array"=w918) -> ("Formatted String"=w916:string)  [unwired: 9 in]
                  n143 = xnode "H5Dread.xnode"("dataset name (this)"="Multiple Decay Fit Parameters SDV Array" ("name"), "error in (no error)"=w870, "default"=w885, "ref in"=w873) -> ("error out"=w889:errorcluster, "data"=w884:dbl[][], "ref out"=w888:T22)  [unwired: 2 in, 1 out]
                  n144 = Array Size(array=w914) -> (size(s)=w915:i32)
                  n145 = Index Array(array=w913) -> (element #1=w912:i32, element #2=w911:i32)  [unwired: 2 in]
                  n146 = Bundle By Name(cluster=w851, "Fit Parameter Constraints"=w894, "Fit Options"=w893, "SYNC Period"=w892, "MLE Baseline Offset Type"=w841, "MLE Baseline Offset"=w840) -> (w891:T1)
                  n147 = Format Into String(format string="Parameter Names: %s\nIRFs Length: %d\n# Data Points: %d x %d", initial string=w921, error in=w889, w916, w915, w912, w911) -> (resulting string=w922:string, error out=w923:errorcluster)
                }
              }
            }
            frame True {
              # "File Type & Version only"
              n148 = call <vilib>:"H5Gclose.vi"("error in (no error)"=w1194, "group in"=w1193) -> ("error out"=w1191:errorcluster)  [unwired: 9 in]
            }
          }
        }
      }
      n149 = call <vilib>:"H5Fclose.vi"("error in (no error)"=w41, "ref"=w42) -> ("error out"=w25:errorcluster)  [unwired: 9 in]
      n150 = call "High Resolution Timing.vi"("relative seconds (NaN)"=w38, "Error In"=w25) -> ("elapsed (relative) seconds"=w37:dbl, "Error Out"=w39:errorcluster)  [unwired: 15 in, 1 out]
    }
  }
  "error out" <- w13
  "elapsed (relative) seconds" <- w6
  "Data Description" <- w4
  "IRFs & Fit Data Map" <- w5
  "Decay Fit Options & Parameters" <- w3
  "[Multiple Decays Fit Parameters SDV]" <- w1
